vi "函数类型4测试.vi"() -> ()   [LabVIEW 2010]
uses:
  全局量/试验配置信息.vi
panel:
  out "合格？":bool[][](array[boolean])
  in  "btn_反选":bool
  out "退出？":bool
  in  "数组_选择":bool[](array[boolean])
  in  "第几组数据":i32
  in  "A_32":bool
  in  "A_31":bool
  in  "A_30":bool
  in  "A_29":bool
  in  "A_28":bool
  in  "A_27":bool
  in  "A_26":bool
  in  "A_25":bool
  in  "A_24":bool
  in  "A_23":bool
  in  "A_22":bool
  in  "A_21":bool
  in  "A_20":bool
  in  "A_19":bool
  in  "A_18":bool
  in  "A_17":bool
  in  "A_16":bool
  in  "A_15":bool
  in  "A_14":bool
  in  "A_13":bool
  in  "A_12":bool
  in  "A_11":bool
  in  "A_10":bool
  in  "A_9":bool
  in  "A_8":bool
  in  "A_7":bool
  in  "A_6":bool
  in  "A_5":bool
  in  "A_4":bool
  in  "A_3":bool
  in  "A_2":bool
  in  "A_1":bool
  in  "btn_全选":bool
  in  "btn_取消":bool
  in  "btn_开始测试":bool
  out "light_32":bool
  out "light_31":bool
  out "light_30":bool
  out "light_29":bool
  out "light_28":bool
  out "light_27":bool
  out "light_26":bool
  out "light_25":bool
  out "light_24":bool
  out "light_23":bool
  out "light_22":bool
  out "light_21":bool
  out "light_20":bool
  out "light_19":bool
  out "light_18":bool
  out "light_17":bool
  out "light_16":bool
  out "light_15":bool
  out "light_14":bool
  out "light_13":bool
  out "light_12":bool
  out "light_11":bool
  out "light_10":bool
  out "light_9":bool
  out "light_8":bool
  out "light_7":bool
  out "light_6":bool
  out "light_5":bool
  out "light_4":bool
  out "light_3":bool
  out "light_2":bool
  out "light_1":bool
  in  "跳变值 2":dbl[](array[numeric])
  in  "跳变值 1":dbl[](array[numeric])
  out "Analog_back":string[][](table) caption="表格"
  in  "Analog_IN":string[][](table) caption="表格"
  # "模拟量输入值（V）"
  # "模拟量反馈值"
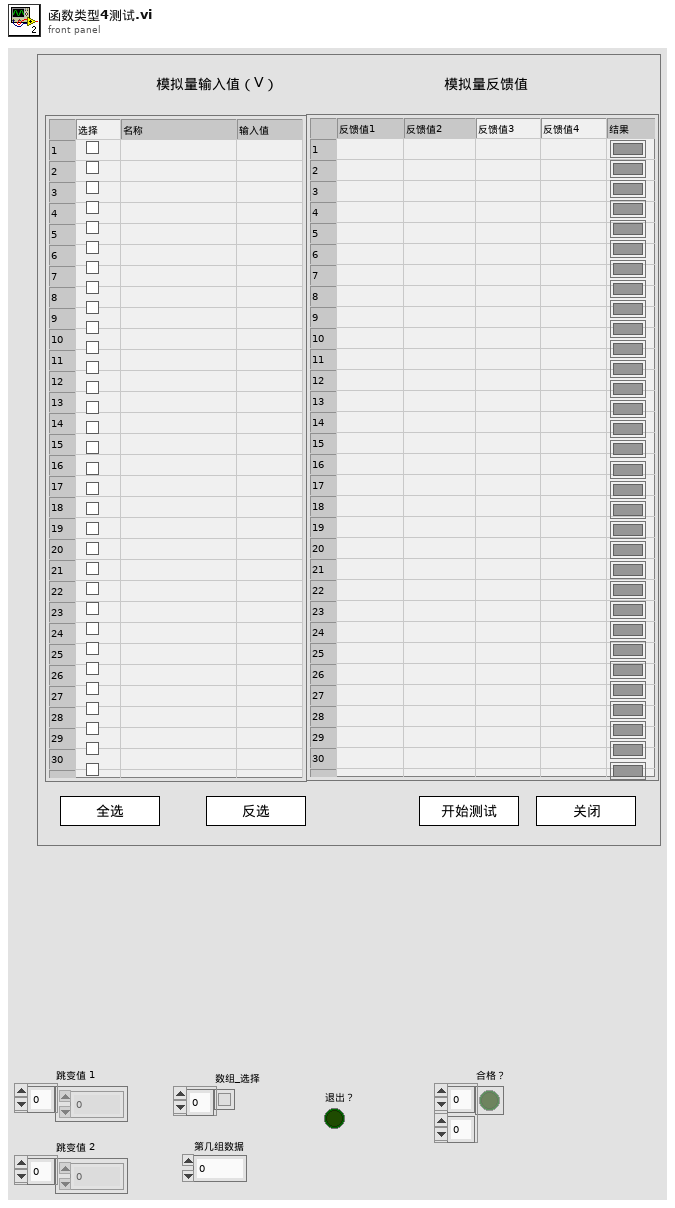
[diagram p1: front panel]
types:
  T1 = enum8{"Enabled", "Disabled", "Disabled and Grayed Out"}
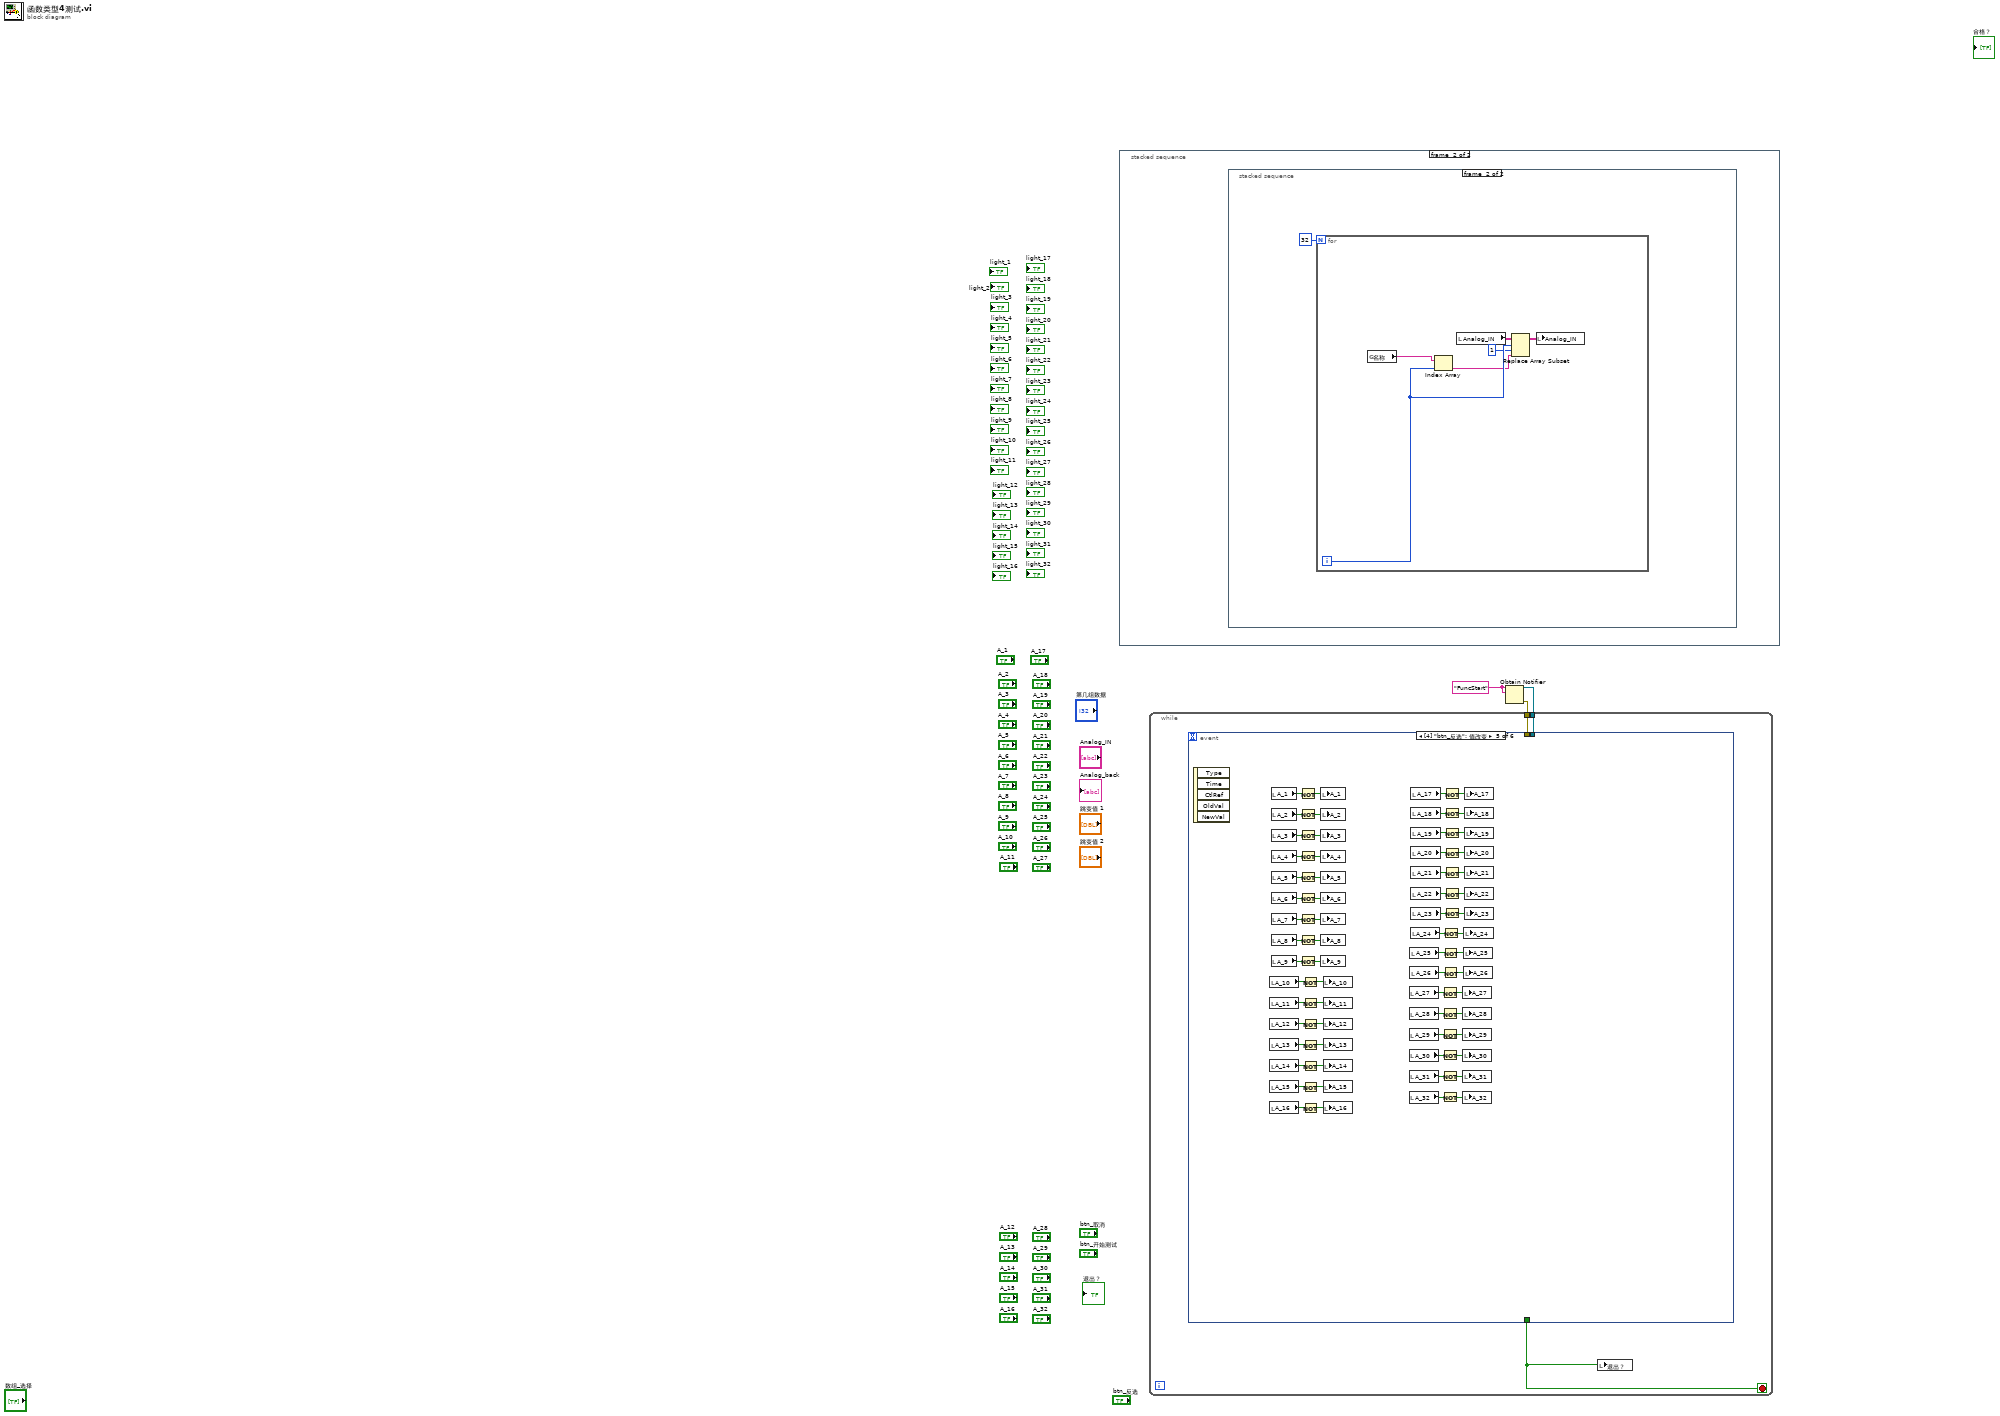
[diagram p0: block diagram]
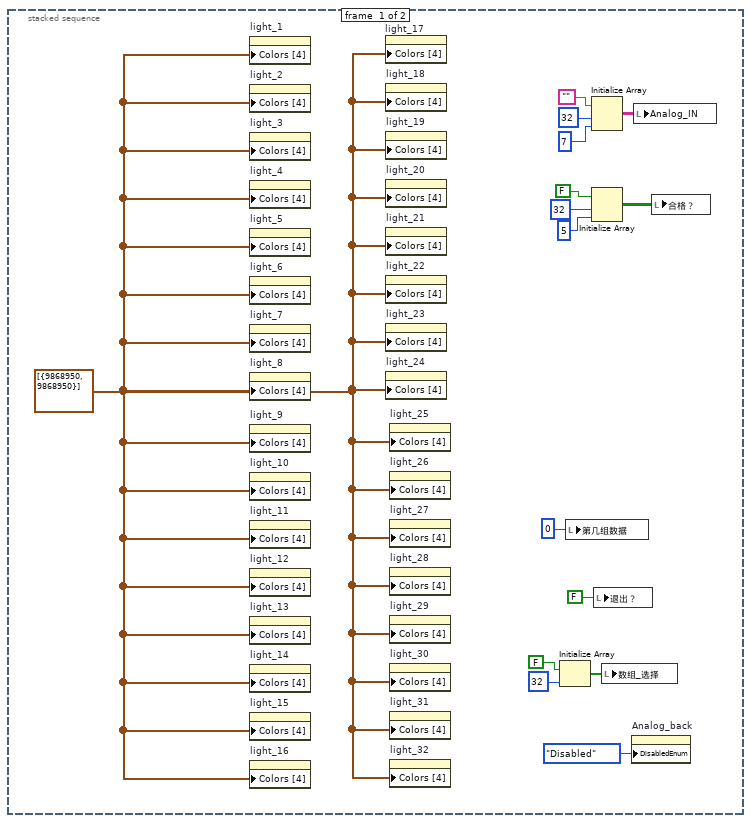
[diagram p2: hidden frame]
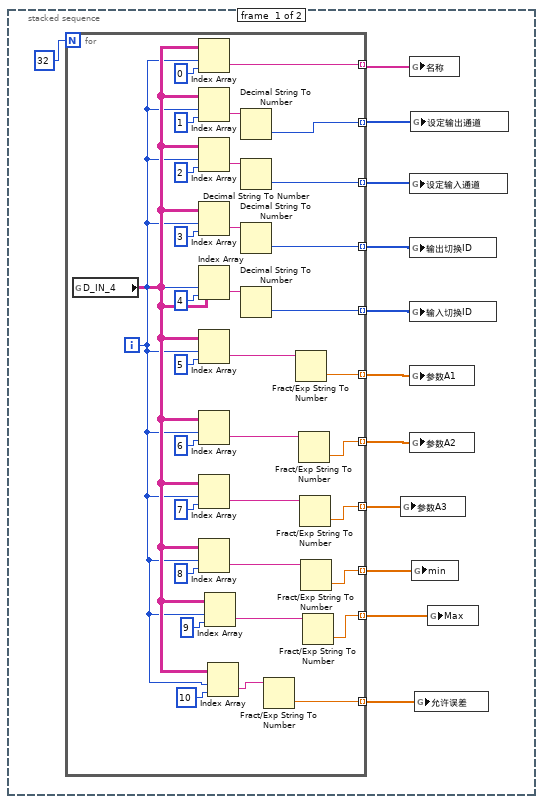
[diagram p3: hidden frame]
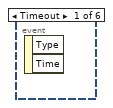
[diagram p4: hidden frame]
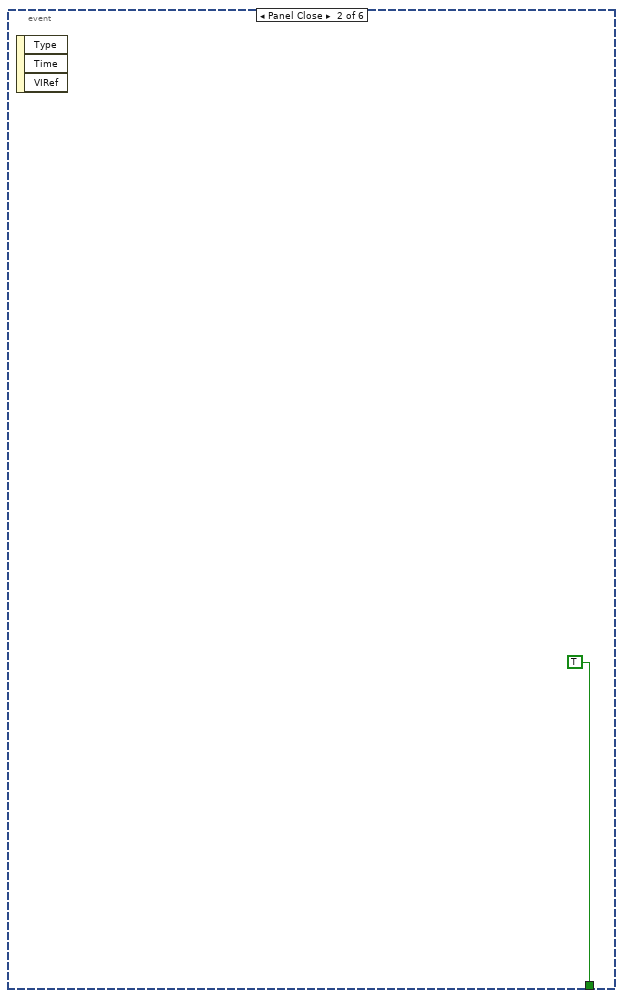
[diagram p5: hidden frame]
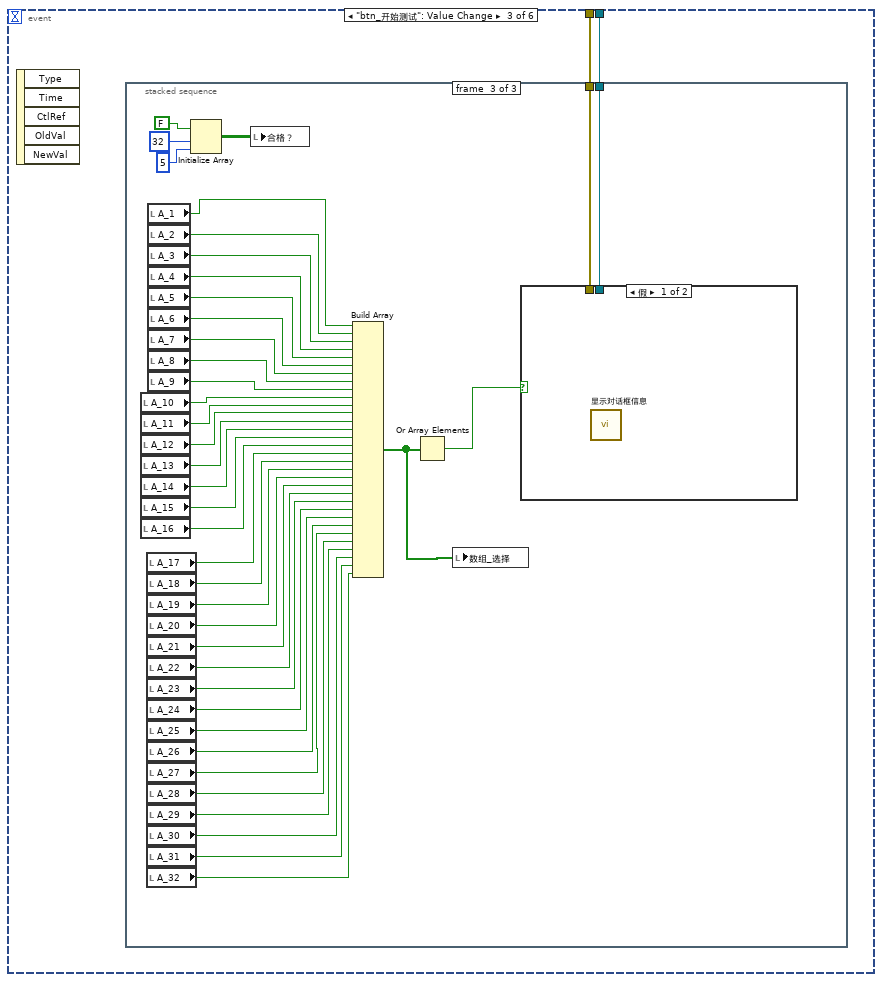
[diagram p6: hidden frame]
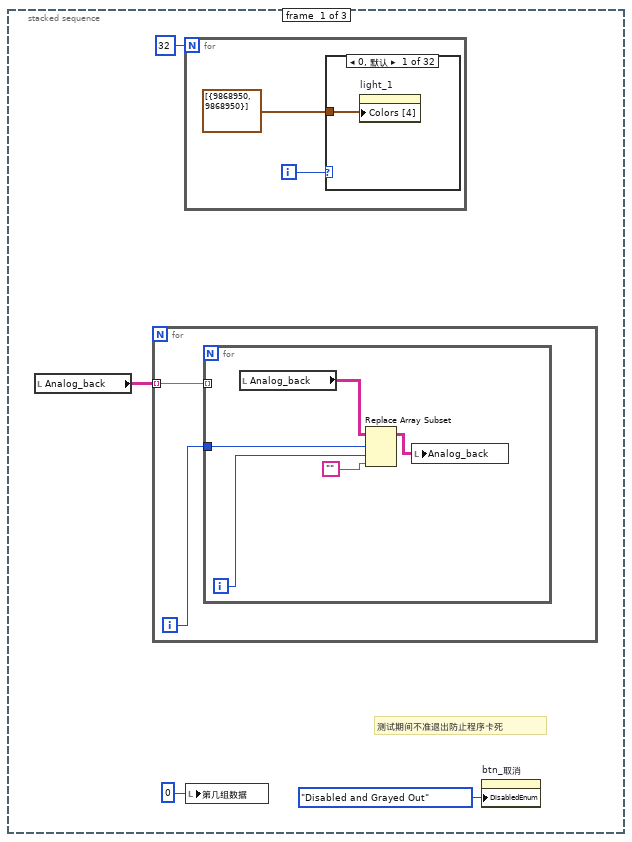
[diagram p7: hidden frame]
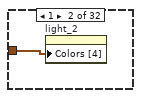
[diagram p8: hidden frame]
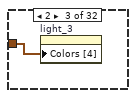
[diagram p9: hidden frame]
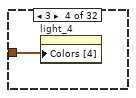
[diagram p10: hidden frame]
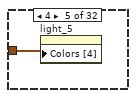
[diagram p11: hidden frame]
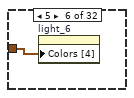
[diagram p12: hidden frame]
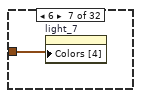
[diagram p13: hidden frame]
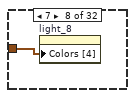
[diagram p14: hidden frame]
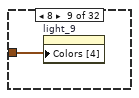
[diagram p15: hidden frame]
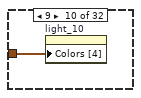
[diagram p16: hidden frame]
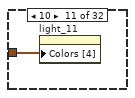
[diagram p17: hidden frame]
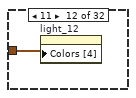
[diagram p18: hidden frame]
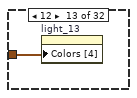
[diagram p19: hidden frame]
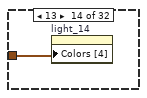
[diagram p20: hidden frame]
diagram:
  w3 = "FuncStart" ("名称（未命名）")
  n1 = stacked-sequence {
    frame #0 {
      w14 = cluster{u32, u32}[] [{9868950, 9868950}]
      n2 = property on="light_1" class="Bool (严格)"("Colors [4]"=w14) -> ()  [unwired: 2 in, 2 out]
      n3 = property on="light_2" class="Bool (严格)"("Colors [4]"=w14) -> ()  [unwired: 2 in, 2 out]
      n4 = property on="light_3" class="Bool (严格)"("Colors [4]"=w14) -> ()  [unwired: 2 in, 2 out]
      n5 = property on="light_4" class="Bool (严格)"("Colors [4]"=w14) -> ()  [unwired: 2 in, 2 out]
      n6 = property on="light_5" class="Bool (严格)"("Colors [4]"=w14) -> ()  [unwired: 2 in, 2 out]
      n7 = property on="light_6" class="Bool (严格)"("Colors [4]"=w14) -> ()  [unwired: 2 in, 2 out]
      n8 = property on="light_7" class="Bool (严格)"("Colors [4]"=w14) -> ()  [unwired: 2 in, 2 out]
      n9 = property on="light_8" class="Bool (严格)"("Colors [4]"=w14) -> ()  [unwired: 2 in, 2 out]
      n10 = property on="light_9" class="Bool (严格)"("Colors [4]"=w14) -> ()  [unwired: 2 in, 2 out]
      n11 = property on="light_10" class="Bool (严格)"("Colors [4]"=w14) -> ()  [unwired: 2 in, 2 out]
      n12 = property on="light_11" class="Bool (严格)"("Colors [4]"=w14) -> ()  [unwired: 2 in, 2 out]
      n13 = property on="light_12" class="Bool (严格)"("Colors [4]"=w14) -> ()  [unwired: 2 in, 2 out]
      n14 = property on="light_13" class="Bool (严格)"("Colors [4]"=w14) -> ()  [unwired: 2 in, 2 out]
      n15 = property on="light_14" class="Bool (严格)"("Colors [4]"=w14) -> ()  [unwired: 2 in, 2 out]
      n16 = property on="light_15" class="Bool (严格)"("Colors [4]"=w14) -> ()  [unwired: 2 in, 2 out]
      n17 = property on="light_16" class="Bool (严格)"("Colors [4]"=w14) -> ()  [unwired: 2 in, 2 out]
      n18 = property on="light_17" class="Bool (严格)"("Colors [4]"=w14) -> ()  [unwired: 2 in, 2 out]
      n19 = property on="light_18" class="Bool (严格)"("Colors [4]"=w14) -> ()  [unwired: 2 in, 2 out]
      n20 = property on="light_19" class="Bool (严格)"("Colors [4]"=w14) -> ()  [unwired: 2 in, 2 out]
      n21 = property on="light_20" class="Bool (严格)"("Colors [4]"=w14) -> ()  [unwired: 2 in, 2 out]
      n22 = property on="light_21" class="Bool (严格)"("Colors [4]"=w14) -> ()  [unwired: 2 in, 2 out]
      n23 = property on="light_22" class="Bool (严格)"("Colors [4]"=w14) -> ()  [unwired: 2 in, 2 out]
      n24 = property on="light_23" class="Bool (严格)"("Colors [4]"=w14) -> ()  [unwired: 2 in, 2 out]
      n25 = property on="light_24" class="Bool (严格)"("Colors [4]"=w14) -> ()  [unwired: 2 in, 2 out]
      n26 = property on="light_25" class="Bool (严格)"("Colors [4]"=w14) -> ()  [unwired: 2 in, 2 out]
      n27 = property on="light_26" class="Bool (严格)"("Colors [4]"=w14) -> ()  [unwired: 2 in, 2 out]
      n28 = property on="light_27" class="Bool (严格)"("Colors [4]"=w14) -> ()  [unwired: 2 in, 2 out]
      n29 = property on="light_28" class="Bool (严格)"("Colors [4]"=w14) -> ()  [unwired: 2 in, 2 out]
      n30 = property on="light_29" class="Bool (严格)"("Colors [4]"=w14) -> ()  [unwired: 2 in, 2 out]
      n31 = property on="light_30" class="Bool (严格)"("Colors [4]"=w14) -> ()  [unwired: 2 in, 2 out]
      n32 = property on="light_31" class="Bool (严格)"("Colors [4]"=w14) -> ()  [unwired: 2 in, 2 out]
      n33 = property on="light_32" class="Bool (严格)"("Colors [4]"=w14) -> ()  [unwired: 2 in, 2 out]
      n34 = Initialize Array(FALSE, 32 ("维数大小")) -> (w12:bool[])
      n35 = local write "第几组数据"(0 ("第几组数据")) -> ()
      n36 = Initialize Array("", 32 ("维数大小"), 7 ("维数大小")) -> (w15:string[][])
      n37 = Initialize Array(FALSE, 32 ("维数大小"), 5 ("维数大小")) -> (w7:bool[][])
      n38 = local write "退出？"(FALSE ("退出？")) -> ()
      n39 = local write "数组_选择"(w12) -> ()
      n40 = property on="Analog_back" class="Tbl (严格)"("DisabledEnum"=T1."Disabled" ("禁用")) -> ()  [unwired: 2 in, 2 out]
      n41 = local write "Analog_IN"(w15) -> ()
      n42 = local write "合格？"(w7) -> ()
    }
    frame #1 {
      n43 = stacked-sequence {
        frame #0 {
          n44 = for {
            N: 32 ("维数大小") -> [_]
            tunnel: [w63] -> w24 mode=indexing
            tunnel: [w59] -> w23 mode=indexing
            tunnel: [w57] -> w22 mode=indexing
            tunnel: [w54] -> w21 mode=indexing
            tunnel: [w51] -> w20 mode=indexing
            tunnel: [w48] -> w26 mode=indexing
            tunnel: [w45] -> w27 mode=indexing
            tunnel: [w42] -> w28 mode=indexing
            tunnel: [w39] -> w29 mode=indexing
            tunnel: [w36] -> w30 mode=indexing
            tunnel: [w31] -> w19 mode=indexing
            i -> [w32]
            n45 = global read "试验配置信息.vi" "D_IN_4"() -> (w33:string[][])
            n46 = Index Array(array=w33, index (row)=w32, index (col)=0 ("禁用的索引 (列)")) -> (element=w63:string)
            n47 = Index Array(array=w33, index (row)=w32, index (col)=1 ("禁用的索引 (列)")) -> (element=w56:string)
            n48 = Index Array(array=w33, index (row)=w32, index (col)=2 ("禁用的索引 (列)")) -> (element=w53:string)
            n49 = Index Array(array=w33, index (row)=w32, index (col)=3 ("禁用的索引 (列)")) -> (element=w49:string)
            n50 = Index Array(array=w33, index (row)=w32, index (col)=4 ("禁用的索引 (列)")) -> (element=w47:string)
            n51 = Index Array(array=w33, index (row)=w32, index (col)=5 ("禁用的索引 (列)")) -> (element=w44:string)
            n52 = Index Array(array=w33, index (row)=w32, index (col)=6 ("禁用的索引 (列)")) -> (element=w40:string)
            n53 = Index Array(array=w33, index (row)=w32, index (col)=7 ("禁用的索引 (列)")) -> (element=w60:string)
            n54 = Index Array(array=w33, index (row)=w32, index (col)=8 ("禁用的索引 (列)")) -> (element=w58:string)
            n55 = Index Array(array=w33, index (row)=w32, index (col)=9 ("禁用的索引 (列)")) -> (element=w37:string)
            n56 = Index Array(array=w33, index (row)=w32, index (col)=10 ("禁用的索引 (列)")) -> (element=w34:string)
            n57 = Decimal String To Number(string=w56) -> (number=w54:i32)  [unwired: 2 in, 1 out]
            n58 = Decimal String To Number(string=w53) -> (number=w51:i32)  [unwired: 2 in, 1 out]
            n59 = Decimal String To Number(string=w49) -> (number=w48:i32)  [unwired: 2 in, 1 out]
            n60 = Decimal String To Number(string=w47) -> (number=w45:i32)  [unwired: 2 in, 1 out]
            n61 = Fract/Exp String To Number(string=w34) -> (number=w31:dbl)  [unwired: 3 in, 1 out]
            n62 = Fract/Exp String To Number(string=w44) -> (number=w42:dbl)  [unwired: 3 in, 1 out]
            n63 = Fract/Exp String To Number(string=w40) -> (number=w39:dbl)  [unwired: 3 in, 1 out]
            n64 = Fract/Exp String To Number(string=w60) -> (number=w59:dbl)  [unwired: 3 in, 1 out]
            n65 = Fract/Exp String To Number(string=w58) -> (number=w57:dbl)  [unwired: 3 in, 1 out]
            n66 = Fract/Exp String To Number(string=w37) -> (number=w36:dbl)  [unwired: 3 in, 1 out]
          }
          n67 = global write "试验配置信息.vi" "参数A3"(w23) -> ()
          n68 = global write "试验配置信息.vi" "名称"(w24) -> ()
          n69 = global write "试验配置信息.vi" "设定输入通道"(w20) -> ()
          n70 = global write "试验配置信息.vi" "输出切换ID"(w26) -> ()
          n71 = global write "试验配置信息.vi" "输入切换ID"(w27) -> ()
          n72 = global write "试验配置信息.vi" "参数A1"(w28) -> ()
          n73 = global write "试验配置信息.vi" "参数A2"(w29) -> ()
          n74 = global write "试验配置信息.vi" "设定输出通道"(w21) -> ()
          n75 = global write "试验配置信息.vi" "min"(w22) -> ()
          n76 = global write "试验配置信息.vi" "允许误差"(w19) -> ()
          n77 = global write "试验配置信息.vi" "Max"(w30) -> ()
        }
        frame #1 {
          n78 = for {
            N: 32 -> [_]
            i -> [w68]
            n79 = global read "试验配置信息.vi" "名称"() -> (w71:string[])
            n80 = Index Array(array=w71, index=w68) -> (element=w67:string)
            n81 = local read "Analog_IN"() -> (w70:string[][])
            n82 = Replace Array Subset(array=w70, new element=w67, index (row)=w68, index (col)=1 ("禁用的索引 (列)")) -> (w69:string[][])
            n83 = local write "Analog_IN"(w69) -> ()
          }
        }
      }
    }
  }
  n84 = Obtain Notifier(name (unnamed)=w3, notification data type=w3) -> (notifier out=w2:refnum<notifier>, error out=w1:errorcluster)  [unwired: 2 in, 1 out]
  n85 = while {
    tunnel: w2 -> [w73]
    tunnel: w1 -> [w72]
    stop <- w74 stop-if-true
    n86 = event shown="[4] \"btn_反选\": 值改变" {
      selector: _ -> [_ _ _ _ _ _]
      dyn-events: _ -> [_ _ _ _ _ _]
      timeout: _ -> [_ _ _ _ _ _]
      tunnel: [_ TRUE _ _ _ TRUE] -> w74
      tunnel: w73 -> [_ _ w77 _ _ _]
      tunnel: w72 -> [_ _ w76 _ _ _]
      event Timeout {
        n87 = event-data() -> ()  [unwired: 1 in, 2 out]
      }
      event Panel Close {
        n88 = event-data() -> ()  [unwired: 1 in, 3 out]
      }
      event "btn_开始测试": Value Change {
        n89 = event-data() -> ()  [unwired: 1 in, 5 out]
        n90 = stacked-sequence {
          tunnel: w77 -> [_ _ w138]
          tunnel: w76 -> [_ _ w137]
          frame #0 {
            # "测试期间不准退出防止程序卡死"
            n91 = local read "Analog_back"() -> (w78:string[][])
            n92 = for {
              tunnel: w78 -> [w83] mode=indexing
              i -> [w82]
              n93 = for {
                tunnel: w83 -> [_] mode=indexing
                tunnel: w82 -> [w85]
                i -> [w84]
                n94 = local read "Analog_back"() -> (w88:string[][])
                n95 = Replace Array Subset(array=w88, new element="", index (row)=w85, index (col)=w84) -> (w87:string[][])
                n96 = local write "Analog_back"(w87) -> ()
              }
            }
            n97 = for {
              N: 32 -> [_]
              i -> [w90]
              n98 = case shown="0, 默认" w90 {
                tunnel: cluster{u32, u32}[] [{9868950, 9868950}] -> [w91 w92 w93 w94 w95 w96 w97 w98 w99 w100 w101 w102 w103 w104 w105 w106 w107 w108 w109 w110 w111 w112 w113 w114 w115 w116 w117 w118 w119 w120 w121 w122]
                frame 0, Default {
                  n99 = property on="light_1" class="Bool (严格)"("Colors [4]"=w91) -> ()  [unwired: 2 in, 2 out]
                }
                frame 1 {
                  n100 = property on="light_2" class="Bool (严格)"("Colors [4]"=w92) -> ()  [unwired: 2 in, 2 out]
                }
                frame 2 {
                  n101 = property on="light_3" class="Bool (严格)"("Colors [4]"=w93) -> ()  [unwired: 2 in, 2 out]
                }
                frame 3 {
                  n102 = property on="light_4" class="Bool (严格)"("Colors [4]"=w94) -> ()  [unwired: 2 in, 2 out]
                }
                frame 4 {
                  n103 = property on="light_5" class="Bool (严格)"("Colors [4]"=w95) -> ()  [unwired: 2 in, 2 out]
                }
                frame 5 {
                  n104 = property on="light_6" class="Bool (严格)"("Colors [4]"=w96) -> ()  [unwired: 2 in, 2 out]
                }
                frame 6 {
                  n105 = property on="light_7" class="Bool (严格)"("Colors [4]"=w97) -> ()  [unwired: 2 in, 2 out]
                }
                frame 7 {
                  n106 = property on="light_8" class="Bool (严格)"("Colors [4]"=w98) -> ()  [unwired: 2 in, 2 out]
                }
                frame 8 {
                  n107 = property on="light_9" class="Bool (严格)"("Colors [4]"=w99) -> ()  [unwired: 2 in, 2 out]
                }
                frame 9 {
                  n108 = property on="light_10" class="Bool (严格)"("Colors [4]"=w100) -> ()  [unwired: 2 in, 2 out]
                }
                frame 10 {
                  n109 = property on="light_11" class="Bool (严格)"("Colors [4]"=w101) -> ()  [unwired: 2 in, 2 out]
                }
                frame 11 {
                  n110 = property on="light_12" class="Bool (严格)"("Colors [4]"=w102) -> ()  [unwired: 2 in, 2 out]
                }
                frame 12 {
                  n111 = property on="light_13" class="Bool (严格)"("Colors [4]"=w103) -> ()  [unwired: 2 in, 2 out]
                }
                frame 13 {
                  n112 = property on="light_14" class="Bool (严格)"("Colors [4]"=w104) -> ()  [unwired: 2 in, 2 out]
                }
                frame 14 {
                  n113 = property on="light_15" class="Bool (严格)"("Colors [4]"=w105) -> ()  [unwired: 2 in, 2 out]
                }
                frame 15 {
                  n114 = property on="light_16" class="Bool (严格)"("Colors [4]"=w106) -> ()  [unwired: 2 in, 2 out]
                }
                frame 16 {
                  n115 = property on="light_17" class="Bool (严格)"("Colors [4]"=w107) -> ()  [unwired: 2 in, 2 out]
                }
                frame 17 {
                  n116 = property on="light_18" class="Bool (严格)"("Colors [4]"=w108) -> ()  [unwired: 2 in, 2 out]
                }
                frame 18 {
                  n117 = property on="light_19" class="Bool (严格)"("Colors [4]"=w109) -> ()  [unwired: 2 in, 2 out]
                }
                frame 19 {
                  n118 = property on="light_20" class="Bool (严格)"("Colors [4]"=w110) -> ()  [unwired: 2 in, 2 out]
                }
                frame 20 {
                  n119 = property on="light_21" class="Bool (严格)"("Colors [4]"=w111) -> ()  [unwired: 2 in, 2 out]
                }
                frame 21 {
                  n120 = property on="light_22" class="Bool (严格)"("Colors [4]"=w112) -> ()  [unwired: 2 in, 2 out]
                }
                frame 22 {
                  n121 = property on="light_23" class="Bool (严格)"("Colors [4]"=w113) -> ()  [unwired: 2 in, 2 out]
                }
                frame 23 {
                  n122 = property on="light_24" class="Bool (严格)"("Colors [4]"=w114) -> ()  [unwired: 2 in, 2 out]
                }
                frame 24 {
                  n123 = property on="light_25" class="Bool (严格)"("Colors [4]"=w115) -> ()  [unwired: 2 in, 2 out]
                }
                frame 25 {
                  n124 = property on="light_26" class="Bool (严格)"("Colors [4]"=w116) -> ()  [unwired: 2 in, 2 out]
                }
                frame 26 {
                  n125 = property on="light_27" class="Bool (严格)"("Colors [4]"=w117) -> ()  [unwired: 2 in, 2 out]
                }
                frame 27 {
                  n126 = property on="light_28" class="Bool (严格)"("Colors [4]"=w118) -> ()  [unwired: 2 in, 2 out]
                }
                frame 28 {
                  n127 = property on="light_29" class="Bool (严格)"("Colors [4]"=w119) -> ()  [unwired: 2 in, 2 out]
                }
                frame 29 {
                  n128 = property on="light_30" class="Bool (严格)"("Colors [4]"=w120) -> ()  [unwired: 2 in, 2 out]
                }
                frame 30 {
                  n129 = property on="light_31" class="Bool (严格)"("Colors [4]"=w121) -> ()  [unwired: 2 in, 2 out]
                }
                frame 31 {
                  n130 = property on="light_32" class="Bool (严格)"("Colors [4]"=w122) -> ()  [unwired: 2 in, 2 out]
                }
              }
            }
            n131 = local write "第几组数据"(0 ("第几组数据")) -> ()
            n132 = property on="btn_取消" class="Bool"("DisabledEnum"=T1."Disabled and Grayed Out" ("禁用")) -> ()  [unwired: 2 in, 2 out]
          }
          frame #1 {
            n133 = for {
              N: 32 -> [_]
              i -> [w125]
              n134 = disable-structure shown="禁用" {
                frame Disabled {
                  n135 = Wait Until Next ms Multiple(millisecond multiple=u32 10 ("毫秒倍数")) -> ()  [unwired: 1 out]
                }
                frame Enabled {
                }
              }
              n136 = for {
                N: 6 -> [_]
                tunnel: w125 -> [w133]
                i -> [w130]
                n137 = Quotient & Remainder(x=w133, y=2) -> (x-y*floor(x/y)=w131:i32)  [unwired: 1 out]
                n138 = Equal To 0?(x=w131) -> (x = 0?=w134:bool)
                n139 = case shown="真" w134 {
                  tunnel: [u32 16448250 u32 15723488] -> w127
                  frame False {
                  }
                  frame True {
                  }
                }
                n140 = Bundle(w133, w130) -> (w129:cluster{i32, i32})  [unwired: 1 in]
                n141 = property on="Analog_back" class="Tbl (严格)"("Active Cell"=w129) -> (error out=w128:errorcluster)  [unwired: 2 in, 1 out]
                n142 = property on="Analog_back" class="Tbl (严格)"(error in=w128, "Cell BG Color"=w127) -> ()  [unwired: 1 in, 2 out]
              }
            }
          }
          frame #2 {
            n143 = local read "A_10"() -> (w162:bool)
            n144 = local read "A_11"() -> (w161:bool)
            n145 = local read "A_12"() -> (w160:bool)
            n146 = local read "A_13"() -> (w159:bool)
            n147 = local read "A_14"() -> (w158:bool)
            n148 = local read "A_15"() -> (w157:bool)
            n149 = local read "A_16"() -> (w156:bool)
            n150 = local read "A_17"() -> (w155:bool)
            n151 = local read "A_18"() -> (w154:bool)
            n152 = local read "A_19"() -> (w153:bool)
            n153 = local read "A_20"() -> (w152:bool)
            n154 = local read "A_21"() -> (w151:bool)
            n155 = local read "A_22"() -> (w150:bool)
            n156 = local read "A_23"() -> (w149:bool)
            n157 = local read "A_24"() -> (w148:bool)
            n158 = local read "A_25"() -> (w147:bool)
            n159 = local read "A_26"() -> (w146:bool)
            n160 = local read "A_27"() -> (w145:bool)
            n161 = local read "A_28"() -> (w144:bool)
            n162 = local read "A_29"() -> (w143:bool)
            n163 = local read "A_30"() -> (w142:bool)
            n164 = local read "A_31"() -> (w141:bool)
            n165 = local read "A_32"() -> (w140:bool)
            n166 = local read "A_1"() -> (w171:bool)
            n167 = local read "A_2"() -> (w170:bool)
            n168 = local read "A_3"() -> (w169:bool)
            n169 = local read "A_4"() -> (w168:bool)
            n170 = local read "A_5"() -> (w167:bool)
            n171 = local read "A_6"() -> (w166:bool)
            n172 = local read "A_7"() -> (w165:bool)
            n173 = local read "A_8"() -> (w164:bool)
            n174 = local read "A_9"() -> (w163:bool)
            n175 = Initialize Array(FALSE, 32 ("维数大小"), 5 ("维数大小")) -> (w173:bool[][])
            n176 = local write "合格？"(w173) -> ()
            n177 = Build Array(w171, w170, w169, w168, w167, w166, w165, w164, w163, w162, w161, w160, w159, w158, w157, w156, w155, w154, w153, w152, w151, w150, w149, w148, w147, w146, w145, w144, w143, w142, w141, w140) -> (w172:bool[])
            n178 = Or Array Elements(Boolean array=w172) -> (logical OR=w139:bool)
            n179 = local write "数组_选择"(w172) -> ()
            n180 = case shown="假" w139 {
              tunnel: w138 -> [_ w178]
              tunnel: w137 -> [_ w177]
              frame False {
                n181 = call "显示对话框信息"() -> ()  [unwired: 10 in, 2 out]
              }
              frame True {
                n182 = Send Notification(notification="start" ("通知"), notifier=w178, error in (no error)=w177) -> ()  [unwired: 2 out]
              }
            }
          }
        }
      }
      event "btn_全选": Value Change {
        w180 = TRUE
        n183 = event-data() -> ()  [unwired: 1 in, 5 out]
        n184 = local write "A_10"(w180) -> ()
        n185 = local write "A_11"(w180) -> ()
        n186 = local write "A_12"(w180) -> ()
        n187 = local write "A_13"(w180) -> ()
        n188 = local write "A_14"(w180) -> ()
        n189 = local write "A_15"(w180) -> ()
        n190 = local write "A_16"(w180) -> ()
        n191 = local write "A_1"(w180) -> ()
        n192 = local write "A_2"(w180) -> ()
        n193 = local write "A_3"(w180) -> ()
        n194 = local write "A_4"(w180) -> ()
        n195 = local write "A_5"(w180) -> ()
        n196 = local write "A_6"(w180) -> ()
        n197 = local write "A_7"(w180) -> ()
        n198 = local write "A_8"(w180) -> ()
        n199 = local write "A_9"(w180) -> ()
        n200 = local write "A_27"(w180) -> ()
        n201 = local write "A_28"(w180) -> ()
        n202 = local write "A_29"(w180) -> ()
        n203 = local write "A_30"(w180) -> ()
        n204 = local write "A_31"(w180) -> ()
        n205 = local write "A_32"(w180) -> ()
        n206 = local write "A_25"(w180) -> ()
        n207 = local write "A_26"(w180) -> ()
        n208 = local write "A_24"(w180) -> ()
        n209 = local write "A_17"(w180) -> ()
        n210 = local write "A_18"(w180) -> ()
        n211 = local write "A_19"(w180) -> ()
        n212 = local write "A_20"(w180) -> ()
        n213 = local write "A_21"(w180) -> ()
        n214 = local write "A_22"(w180) -> ()
        n215 = local write "A_23"(w180) -> ()
      }
      event "btn_反选": Value Change {
        n216 = event-data() -> ()  [unwired: 1 in, 5 out]
        n217 = local read "A_10"() -> (w231:bool)
        n218 = local read "A_11"() -> (w230:bool)
        n219 = local read "A_12"() -> (w229:bool)
        n220 = local read "A_13"() -> (w228:bool)
        n221 = local read "A_14"() -> (w227:bool)
        n222 = local read "A_15"() -> (w226:bool)
        n223 = local read "A_16"() -> (w225:bool)
        n224 = local read "A_1"() -> (w244:bool)
        n225 = local read "A_2"() -> (w242:bool)
        n226 = local read "A_3"() -> (w240:bool)
        n227 = local read "A_4"() -> (w237:bool)
        n228 = local read "A_5"() -> (w236:bool)
        n229 = local read "A_6"() -> (w235:bool)
        n230 = local read "A_7"() -> (w234:bool)
        n231 = local read "A_8"() -> (w233:bool)
        n232 = local read "A_9"() -> (w232:bool)
        n233 = Not(x=w244) -> (.not. x?=w243:bool)
        n234 = Not(x=w242) -> (.not. x?=w241:bool)
        n235 = Not(x=w240) -> (.not. x?=w239:bool)
        n236 = Not(x=w237) -> (.not. x?=w238:bool)
        n237 = Not(x=w236) -> (.not. x?=w224:bool)
        n238 = Not(x=w235) -> (.not. x?=w223:bool)
        n239 = Not(x=w234) -> (.not. x?=w222:bool)
        n240 = Not(x=w233) -> (.not. x?=w221:bool)
        n241 = Not(x=w232) -> (.not. x?=w220:bool)
        n242 = Not(x=w231) -> (.not. x?=w219:bool)
        n243 = Not(x=w230) -> (.not. x?=w218:bool)
        n244 = Not(x=w229) -> (.not. x?=w217:bool)
        n245 = Not(x=w228) -> (.not. x?=w216:bool)
        n246 = Not(x=w227) -> (.not. x?=w215:bool)
        n247 = Not(x=w226) -> (.not. x?=w214:bool)
        n248 = Not(x=w225) -> (.not. x?=w213:bool)
        n249 = local write "A_1"(w243) -> ()
        n250 = local write "A_2"(w241) -> ()
        n251 = local write "A_3"(w239) -> ()
        n252 = local write "A_4"(w238) -> ()
        n253 = local write "A_5"(w224) -> ()
        n254 = local write "A_6"(w223) -> ()
        n255 = local write "A_7"(w222) -> ()
        n256 = local write "A_8"(w221) -> ()
        n257 = local write "A_9"(w220) -> ()
        n258 = local write "A_10"(w219) -> ()
        n259 = local write "A_11"(w218) -> ()
        n260 = local write "A_12"(w217) -> ()
        n261 = local write "A_13"(w216) -> ()
        n262 = local write "A_14"(w215) -> ()
        n263 = local write "A_15"(w214) -> ()
        n264 = local write "A_16"(w213) -> ()
        n265 = local read "A_27"() -> (w191:bool)
        n266 = local read "A_28"() -> (w189:bool)
        n267 = local read "A_29"() -> (w187:bool)
        n268 = local read "A_30"() -> (w185:bool)
        n269 = local read "A_31"() -> (w183:bool)
        n270 = local read "A_32"() -> (w181:bool)
        n271 = local read "A_25"() -> (w195:bool)
        n272 = local read "A_26"() -> (w193:bool)
        n273 = local read "A_24"() -> (w197:bool)
        n274 = local read "A_17"() -> (w211:bool)
        n275 = local read "A_18"() -> (w209:bool)
        n276 = local read "A_19"() -> (w207:bool)
        n277 = local read "A_20"() -> (w205:bool)
        n278 = local read "A_21"() -> (w202:bool)
        n279 = local read "A_22"() -> (w201:bool)
        n280 = local read "A_23"() -> (w198:bool)
        n281 = Not(x=w191) -> (.not. x?=w190:bool)
        n282 = Not(x=w189) -> (.not. x?=w188:bool)
        n283 = Not(x=w187) -> (.not. x?=w186:bool)
        n284 = Not(x=w185) -> (.not. x?=w184:bool)
        n285 = Not(x=w183) -> (.not. x?=w182:bool)
        n286 = Not(x=w181) -> (.not. x?=w212:bool)
        n287 = Not(x=w195) -> (.not. x?=w194:bool)
        n288 = Not(x=w193) -> (.not. x?=w192:bool)
        n289 = Not(x=w197) -> (.not. x?=w196:bool)
        n290 = Not(x=w211) -> (.not. x?=w210:bool)
        n291 = Not(x=w209) -> (.not. x?=w208:bool)
        n292 = Not(x=w207) -> (.not. x?=w206:bool)
        n293 = Not(x=w205) -> (.not. x?=w204:bool)
        n294 = Not(x=w202) -> (.not. x?=w203:bool)
        n295 = Not(x=w201) -> (.not. x?=w200:bool)
        n296 = Not(x=w198) -> (.not. x?=w199:bool)
        n297 = local write "A_27"(w190) -> ()
        n298 = local write "A_28"(w188) -> ()
        n299 = local write "A_29"(w186) -> ()
        n300 = local write "A_30"(w184) -> ()
        n301 = local write "A_31"(w182) -> ()
        n302 = local write "A_32"(w212) -> ()
        n303 = local write "A_25"(w194) -> ()
        n304 = local write "A_26"(w192) -> ()
        n305 = local write "A_24"(w196) -> ()
        n306 = local write "A_17"(w210) -> ()
        n307 = local write "A_18"(w208) -> ()
        n308 = local write "A_19"(w206) -> ()
        n309 = local write "A_20"(w204) -> ()
        n310 = local write "A_21"(w203) -> ()
        n311 = local write "A_22"(w200) -> ()
        n312 = local write "A_23"(w199) -> ()
      }
      event "btn_取消": Value Change {
        n313 = event-data() -> ()  [unwired: 1 in, 5 out]
      }
    }
    n314 = local write "退出？"(w74) -> ()
  }
